vi "MGI Center from 3 Points (DBL).vi"(1 "Three Points":dbl[][](array[numeric])=[[0.0, 0.0, 0.0], [0.0, 0.0, 0.0], [0.0, 0.0, 0.0]] format="%_7g") -> (0 "Center":dbl[](array[numeric]) format="%#_7g")   [LabVIEW 2020]
doc: "Calculate the center of a circle based on three points on the circle. \n\nAuthored by David A. Moore\nsupport@mooregoodideas.com\nwww.mooregoodideas.com\n\nCopyright (c) 2010, Moore Good Ideas, Inc.\n\nAll rights reserved.\n\nRedistribution and use in source and binary forms, with or without modification, are permitted provided that the following conditions are met:\n\n * Redistributions of source code must retain the above copyright notice, this list of conditions and the following disclaimer.\n * Redistributions in binary form must reproduce the above copyright notice, this list of conditions and the following disclaimer in the documentation and/or other materials provided with the distribution.\n * Neither the name of Moore Good Ideas, Inc. nor the names of its contributors may be used to endorse or promote products derived from this software without specific prior written permission.\n\nTHIS SOFTWARE IS PROVIDED BY THE COPYRIGHT HOLDERS AND CONTRIBUTORS \"AS IS\" AND ANY EXPRESS OR IMPLIED WARRANTIES, INCLUDING, BUT NOT LIMITED TO, THE IMPLIED WARRANTIES OF MERCHANTABILITY AND FITNESS FOR A PARTICULAR PURPOSE ARE DISCLAIMED. IN NO EVENT SHALL THE COPYRIGHT OWNER OR CONTRIBUTORS BE LIABLE FOR ANY DIRECT, INDIRECT, INCIDENTAL, SPECIAL, EXEMPLARY, OR CONSEQUENTIAL DAMAGES (INCLUDING, BUT NOT LIMITED TO, PROCUREMENT OF SUBSTITUTE GOODS OR SERVICES; LOSS OF USE, DATA, OR PROFITS; OR BUSINESS INTERRUPTION) HOWEVER CAUSED AND ON ANY THEORY OF LIABILITY, WHETHER IN CONTRACT, STRICT LIABILITY, OR TORT (INCLUDING NEGLIGENCE OR OTHERWISE) ARISING IN ANY WAY OUT OF THE USE OF THIS SOFTWARE, EVEN IF ADVISED OF THE POSSIBILITY OF SUCH DAMAGE."
uses:
  <userlib>/_MGI/Matrix & Vector/MGI Calculate Vector Length/MGI Calculate Vector Length DBL.vi
  <userlib>/_MGI/Matrix & Vector/MGI Dot Product/MGI Dot Product DBL.vi
panel:
  # "y"
  # "x"
  # "z"
  # "y"
  # "z"
  # "x"
  # "p1"
  # "p2"
  # "p3"
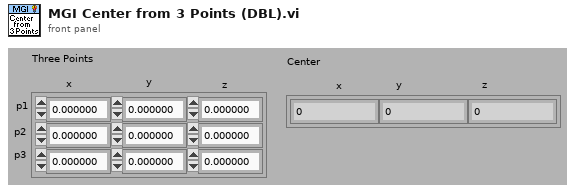
[diagram p1: front panel]
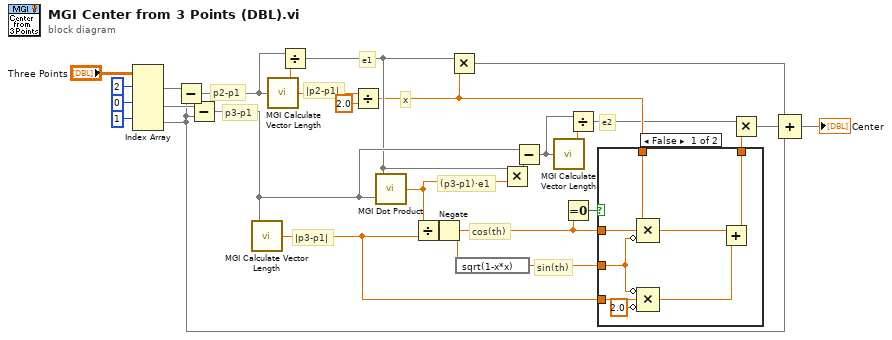
[diagram p0: block diagram]
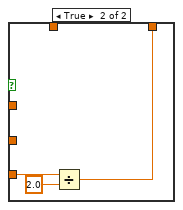
[diagram p2: hidden frame]
diagram:
  # "x"
  # "e2"
  # "sin(th)"
  # "cos(th)"
  # "(p3-p1)·e1"
  # "|p3-p1|"
  # "|p2-p1|"
  # "p3-p1"
  # "p2-p1"
  # "e1"
  n1 = Index Array(array="Three Points", index (row) #1=2 ("index (row)"), index (row) #2=0 ("index (row)"), index (row) #3=1 ("index (row)")) -> (element #1=w23:dbl[], element #2=w21:dbl[], element #3=w5:dbl[])  [unwired: 3 in]
  n2 = Subtract(x=w23, y=w5) -> (x-y=w22:dbl[])
  n3 = Subtract(x=w21, y=w5) -> (x-y=w17:dbl[])
  n4 = call-poly <userlib>:"MGI Calculate Vector Length.vi"("Vector"=w17) -> ("Distance"=w12:dbl)
  n5 = call-poly <userlib>:"MGI Calculate Vector Length.vi"("Vector"=w22) -> ("Distance"=w20:dbl)
  n6 = Divide(x=w22, y=w20) -> (x/y=w13:dbl[])
  n7 = Divide(x=w20, y=sgl 2.0) -> (x/y=w11:dbl)
  n8 = call-poly <userlib>:"MGI Dot Product.vi"("Y Vector"=w17, "X Vector"=w13) -> ("X * Y"=w14:dbl)
  n9 = Divide(x=w14, y=w12) -> (x/y=w2:dbl)
  n10 = Negate(x=w2) -> (-x=w1:dbl)
  n11 = Multiply(x=w13, y=w11) -> (x*y=w6:dbl[])
  n12 = expression code="sqrt(1-x*x)"(w1) -> (w10:dbl)
  n13 = Multiply(x=w13, y=w14) -> (x*y=w18:dbl[])
  n14 = Subtract(x=w17, y=w18) -> (x-y=w15:dbl[])
  n15 = call-poly <userlib>:"MGI Calculate Vector Length.vi"("Vector"=w15) -> ("Distance"=w16:dbl)
  n16 = Equal To 0?(x=w1) -> (x = 0?=w3:bool)
  n17 = Divide(x=w15, y=w16) -> (x/y=w9:dbl[])
  n18 = case shown="False" w3 {
    tunnel: w12 -> [w35 w38]
    tunnel: w11 -> [w33 _]
    tunnel: w1 -> [w32 _]
    tunnel: w10 -> [w31 _]
    tunnel: [w28 w36] -> w8
    frame False {
      n19 = Compound Arithmetic op=MULTIPLY(w33, w32, invert w31) -> (w30:dbl)
      n20 = Compound Arithmetic op=MULTIPLY(invert w31, w35, invert 2.0 ("value")) -> (w29:dbl)
      n21 = Add(x=w30, y=w29) -> (x+y=w28:dbl)
    }
    frame True {
      n22 = Divide(x=w38, y=2.0) -> (x/y=w36:dbl)
    }
  }
  n23 = Multiply(x=w9, y=w8) -> (x*y=w7:dbl[])
  n24 = Compound Arithmetic op=ADD(w6, w7, w5) -> (→"Center":dbl[])
